vi "oa_SCL Draw Sized Squares.vi"(6 "multi-color(F)":bool, 8 "color(yellow)":u32(colorbox)=16776960, 9 "sized scatter plot cosmetics":T1={"min size"=1, "max size"=5, "maps to max size"=5, "color array"=[16776960, 65280, 16711680, 255]}, 10 "data":cluster{"x":i16, "y":i16, "c":i16}[](array[cluster]), 11 "picture":picture) -> (3 "new picture":picture)   [LabVIEW 2017]
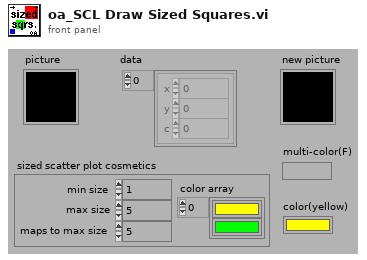
[diagram p1: front panel]
types:
  T1 = cluster{"min size":i16, "max size":i16, "maps to max size":i16, "color array":u32[]}
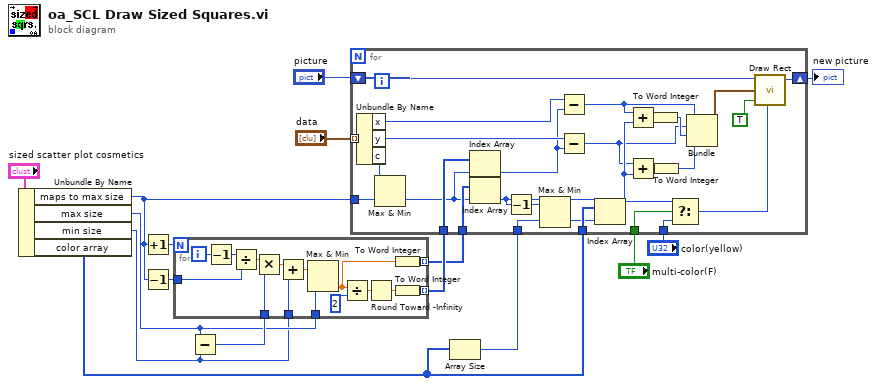
[diagram p0: block diagram]
diagram:
  n1 = Unbundle By Name("sized scatter plot cosmetics") -> ("maps to max size"=w7:i16, "max size"=w6:i16, "min size"=w5:i16, "color array"=w2:u32[])
  n2 = Increment(x=w7) -> (x+1=w9:i16)
  n3 = Decrement(x=w7) -> (x-1=w10:i16)
  n4 = Subtract(x=w6, y=w5) -> (x-y=w11:i16)
  n5 = for {
    N: w9 -> [_]
    tunnel: w5 -> [w27]
    tunnel: w10 -> [w23]
    tunnel: [w20] -> w13 mode=indexing
    tunnel: w6 -> [w26]
    tunnel: [w21] -> w12 mode=indexing
    tunnel: w11 -> [w24]
    i -> [w28]
    n6 = Decrement(x=w28) -> (x-1=w22:i32)
    n7 = Divide(x=w22, y=w23) -> (x/y=w29:dbl)
    n8 = Multiply(x=w29, y=w24) -> (x*y=w31:dbl)
    n9 = Add(x=w31, y=w27) -> (x+y=w25:dbl)
    n10 = Max & Min(x=w25, y=w26) -> (min(x,y)=w19:dbl)  [unwired: 1 out]
    n11 = Divide(x=w19, y=2) -> (x/y=w18:dbl)
    n12 = Round Toward -Infinity(1:w18) -> (0:w17:dbl)
    n13 = To Word Integer(number=w19) -> (16bit integer=w21:i16)
    n14 = To Word Integer(number=w17) -> (16bit integer=w20:i16)
  }
  n15 = Array Size(array=w2) -> (size(s)=w1:i32)
  n16 = for {
    tunnel: "data" -> [w56] mode=indexing
    shift-right: [w57] -> w14
    shift-left: "picture" -> [w58]
    tunnel: w2 -> [w41]
    tunnel: w13 -> [w48]
    tunnel: w12 -> [w47]
    tunnel: w7 -> [w44]
    tunnel: "multi-color(F)" -> [w39]
    tunnel: "color(yellow)" -> [w37]
    tunnel: w1 -> [w32]
    n17 = Unbundle By Name(w56) -> ("x"=w53:i16, "y"=w54:i16, "c"=w45:i16)
    n18 = Max & Min(x=w45, y=w44) -> (min(x,y)=w43:i16)  [unwired: 1 out]
    n19 = Index Array(array=w48, index=w43) -> (element=w46:i16)
    n20 = Index Array(array=w47, index=w43) -> (element=w59:i16)
    n21 = Decrement(x=w59) -> (x-1=w33:i16)
    n22 = Max & Min(x=w33, y=w32) -> (min(x,y)=w34:i32)  [unwired: 1 out]
    n23 = Subtract(x=w53, y=w46) -> (x-y=w36:i16)
    n24 = Subtract(x=w54, y=w46) -> (x-y=w35:i16)
    n25 = Index Array(array=w41, index=w34) -> (element=w38:u32)
    n26 = Add(x=w36, y=w59) -> (x+y=w51:i16)
    n27 = Add(x=w35, y=w59) -> (x+y=w52:i16)
    n28 = To Word Integer(number=w51) -> (16bit integer=w49:i16)
    n29 = To Word Integer(number=w52) -> (16bit integer=w50:i16)
    n30 = Select(t=w38, s=w39, f=w37) -> (s? t:f=w40:u32)
    n31 = Bundle(w36, w35, w49, w50) -> (w42:cluster{i16, i16, i16, i16})  [unwired: 1 in]
    n32 = call <vilib>:"Draw Rect.vi"("picture"=w58, "rect"=w42, "fill?(F)"=TRUE, "color(black)"=w40) -> ("new picture"=w57:picture)  [unwired: 5 in]
  }
  "new picture" <- w14
